vi "Matthews_Corrcoef.vi"(8 "error in (no error)":errorcluster caption="entrée d'erreur (pas d'erreur)", 9 "y_pred":string[][](array[string]), 10 "y_true":string[][](array[string]), 11 "matthews_corrcoef":cluster{"sample_weight":dbl[]}) -> (0 "error out":errorcluster caption="sortie d'erreur", 3 "Score":string)   [LabVIEW 2020]
doc: "Compute the Matthews correlation coefficient (MCC)\n\nThe Matthews correlation coefficient is used in machine learning as a measure of the quality of binary and multiclass classifications. It takes into account true and false positives and negatives and is generally regarded as a balanced measure which can be used even if the classes are of very different sizes. The MCC is in essence a correlation coefficient value between -1 and +1. A coefficient of +1 represents a perfect prediction, 0 an average random prediction and -1 an inverse prediction. The statistic is also known as the phi coefficient. [source: Wikipedia]\n\nBinary and multiclass labels are supported. Only in the binary case does this relate to information about true and false positives and negatives. See references below.\n\n\n\nParameters : \n\n- y_true : array, shape = [n_samples]\nGround truth (correct) target values.\n\n- y_pred : array, shape = [n_samples]\nEstimated targets as returned by a classifier.\n\n- sample_weight : array-like of shape (n_samples,), default=None\nSample weights.\n\nReturns : \n\n- mcc : float\nThe Matthews correlation coefficient (+1 represents a perfect prediction, 0 an average random prediction and -1 and inverse prediction)."
uses:
  Matthews_Corrcoef.lvclass
panel:
  out "Matthews_Corrcoef.lvclass":refnum<class "Matthews_Corrcoef.lvclass">
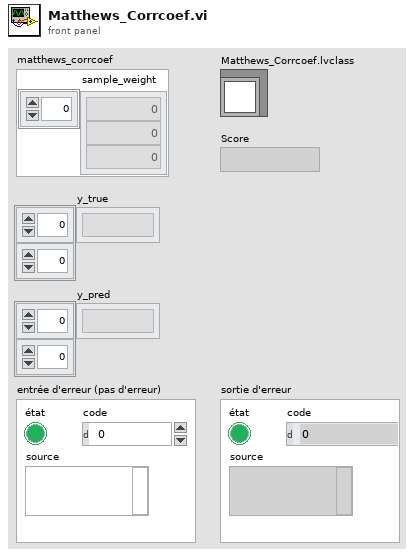
[diagram p1: front panel]
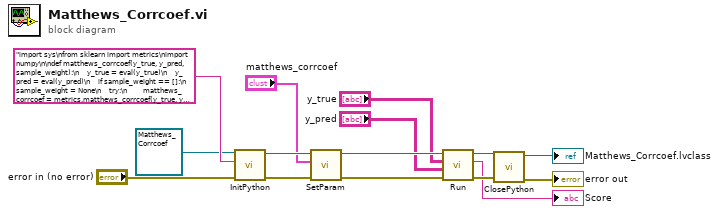
[diagram p0: block diagram]
diagram:
  n1 = call-dynamic "InitPython.vi"("error in (no error)"="error in (no error)", "Python Instruction"="import sys\nfrom sklearn import metrics\nimport numpy\n\ndef matthews_corrcoef(y_true, y_pred, sample_weight):\n    y_true = eval(y_true)\n    y_pred = eval(y_pred)\n    if sample_weight == []:\n        sample_weight = None\n    try:\n        matthews_corrcoef = metrics.matthews_corrcoef(y_true, y_pred, sample_weight)\n        matthews_corrcoef = matthews_corrcoef.tolist()\n        return str(matthews_corrcoef)\n    except:\n        erreur = sys.exc_info()\n        typerr = u\"%s\" % (erreur[0])\n        typerr = typerr[typerr.find(\"'\")+1:typerr.rfind(\"'\")]\n        msgerr = u\"%s\" % (erreur[1])\n        message = str('/!\\\\ {0} : {1}'. format(typerr,msgerr))\n        return message", "Scikit-learn en entrée"=refnum<class "Matthews_Corrcoef.lvclass"> refnum ("Matthews_Corrcoef.lvclass")) -> ("error out"=w11:errorcluster, "Scikit-learn en sortie"=w10:refnum<class "Matthews_Corrcoef.lvclass">)  [unwired: 7 in]
  n2 = call-dynamic "SetParam.vi"("error in (no error)"=w11, "matthews_corrcoef"="matthews_corrcoef", "Matthews_Corrcoef.lvclass"=w10) -> ("error out"=w7:errorcluster, "Matthews_Corrcoef.lvclass"=w8:refnum<class "Matthews_Corrcoef.lvclass">)  [unwired: 7 in]
  n3 = call-dynamic "Run.vi"("error in (no error)"=w7, "y_pred"="y_pred", "y_true"="y_true", "Matthews_Corrcoef.lvclass"=w8) -> ("error out"=w5:errorcluster, "String Data"=→"Score":string, "Matthews_Corrcoef.lvclass"=w6:refnum<class "Matthews_Corrcoef.lvclass">)  [unwired: 5 in]
  n4 = call-dynamic "ClosePython.vi"("error in (no error)"=w5, "Scikit-learn en entrée"=w6) -> ("error out"=→"error out":errorcluster, "Scikit-learn en sortie"=→"Matthews_Corrcoef.lvclass":refnum<class "Matthews_Corrcoef.lvclass">)  [unwired: 8 in]
